vi "WT230.vi"(7 "simulazione":bool, 8 "error in (no error)":errorcluster, 11 "Queue Name":string="WT230_Q") -> (0 "error out":errorcluster, 2 "Stopped":bool)   [LabVIEW 2019]
uses:
  TypeDef/MISURE WT.ctl
  TypeDef/DEVICE NAME.ctl
  <vilib>/Utility/file.llb/Read From Spreadsheet File (string).vi
  <vilib>/Instr/_visa.llb/VISA Configure Serial Port (Instr).vi
  Globals.vi
panel:
  out "String 2":string
  out "error out 3":errorcluster
  out "error out 2":errorcluster
  out "Numeric":i32
  out "String":string
  out "WT230 CONFIG":string[][](array[string])
  out "MISURE WT":T1
  in  "write buffer":string=":MEAS:NORM:ITEM:V:ELEM1 1;ELEM2 1;ELEM3 1;SIGMA 1;:MEAS:NORM:ITEM:A:ELEM1 1;ELEM2 1;ELEM3 1;SIGMA 1;:MEAS:NORM:ITEM:W:ELEM1 1;ELEM2 1;ELEM3 1;SIGMA 1;:MEAS:NORM:ITEM:VA:ELEM1 1;:MEAS:NORM:ITEM:PF:ELEM1 1;:MEAS:NORM:ITEM:PF:SIGMA 1;:MEAS:NORM:ITEM:VHZ:ELEM1 1;"
  out "# elements in queue":i32
  out "Inizialize error":errorcluster
  out "WT230 Settings":string[][](array[string])
  out "LOOP TIME (ms)":u32
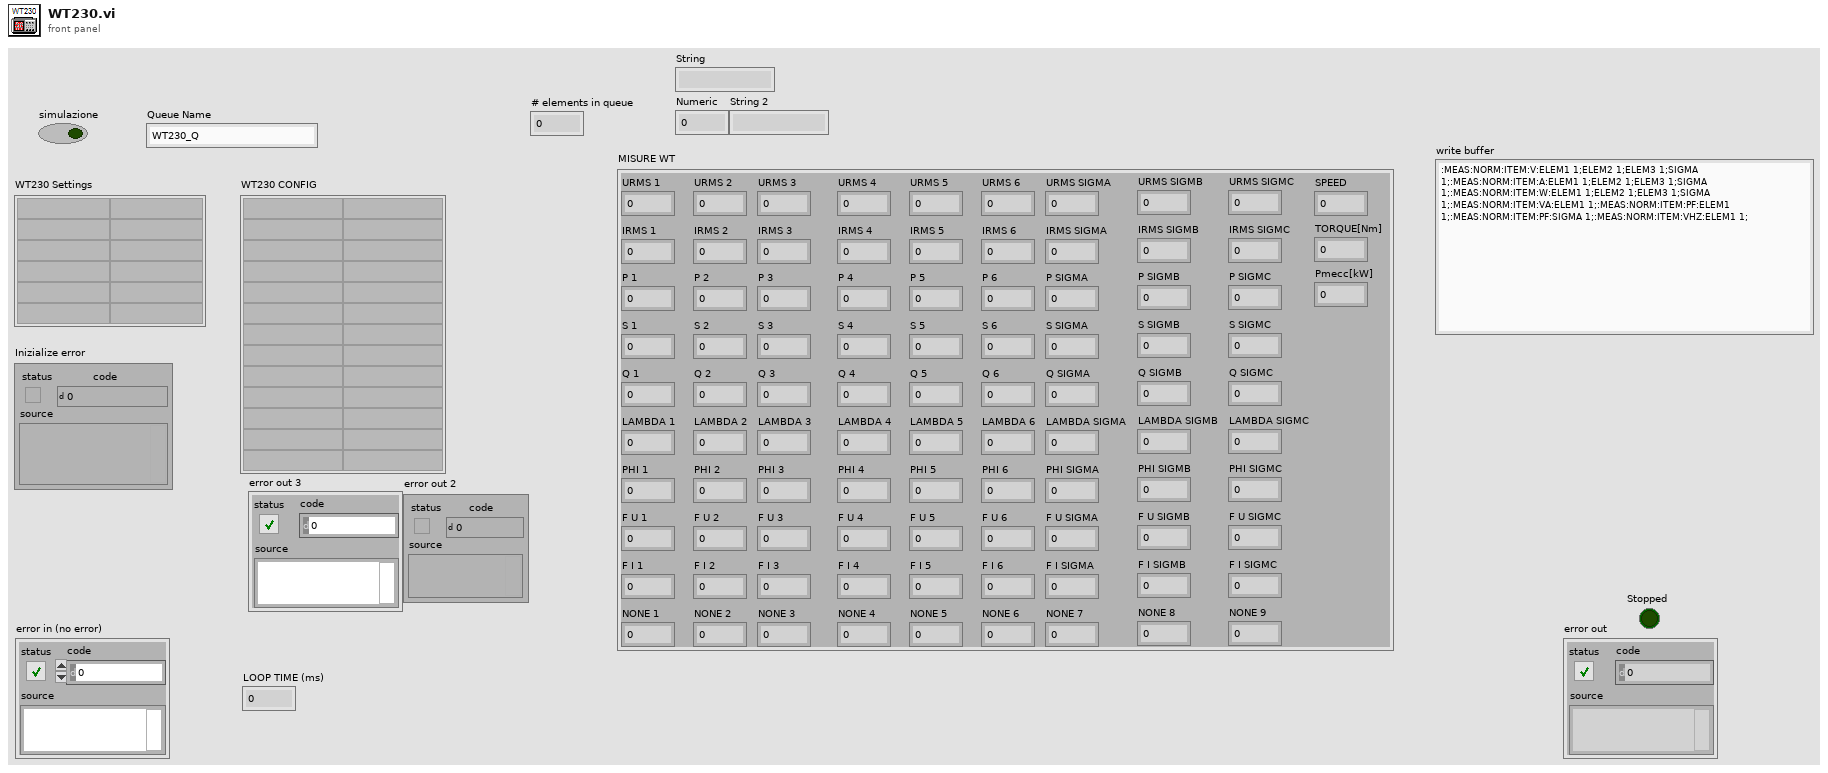
[diagram p1: front panel]
types:
  T1 = typedef "MISURE WT.ctl" = cluster{"URMS 1":dbl, "IRMS 1":dbl, "P 1":dbl, "S 1":dbl, "Q 1":dbl, "LAMBDA 1":dbl, "PHI 1":dbl, "F U 1":dbl, "F I 1":dbl, "NONE 1":dbl, "URMS 2":dbl, "IRMS 2":dbl, "P 2":dbl, "S 2":dbl, "Q 2":dbl, "LAMBDA 2":dbl, "PHI 2":dbl, "F U 2":dbl, "F I 2":dbl, "NONE 2":dbl, "URMS 3":dbl, "IRMS 3":dbl, "P 3":dbl, "S 3":dbl, "Q 3":dbl, "LAMBDA 3":dbl, "PHI 3":dbl, "F U 3":dbl, "F I 3":dbl, "NONE 3":dbl, "URMS 4":dbl, "IRMS 4":dbl, "P 4":dbl, "S 4":dbl, "Q 4":dbl, "LAMBDA 4":dbl, "PHI 4":dbl, "F U 4":dbl, "F I 4":dbl, "NONE 4":dbl, "URMS 5":dbl, "IRMS 5":dbl, "P 5":dbl, "S 5":dbl, "Q 5":dbl, "LAMBDA 5":dbl, "PHI 5":dbl, "F U 5":dbl, "F I 5":dbl, "NONE 5":dbl, "URMS 6":dbl, "IRMS 6":dbl, "P 6":dbl, "S 6":dbl, "Q 6":dbl, "LAMBDA 6":dbl, "PHI 6":dbl, "F U 6":dbl, "F I 6":dbl, "NONE 6":dbl, "URMS SIGMA":dbl, "IRMS SIGMA":dbl, "P SIGMA":dbl, "S SIGMA":dbl, "Q SIGMA":dbl, "LAMBDA SIGMA":dbl, "PHI SIGMA":dbl, "F U SIGMA":dbl, "F I SIGMA":dbl, "NONE 7":dbl, "URMS SIGMB":dbl, "IRMS SIGMB":dbl, "P SIGMB":dbl, "S SIGMB":dbl, "Q SIGMB":dbl, "LAMBDA SIGMB":dbl, "PHI SIGMB":dbl, "F U SIGMB":dbl, "F I SIGMB":dbl, "NONE 8":dbl, "URMS SIGMC":dbl, "IRMS SIGMC":dbl, "P SIGMC":dbl, "S SIGMC":dbl, "Q SIGMC":dbl, "LAMBDA SIGMC":dbl, "PHI SIGMC":dbl, "F U SIGMC":dbl, "F I SIGMC":dbl, "NONE 9":dbl, "SPEED":dbl, "TORQUE[Nm]":dbl, "Pmecc[kW]":dbl}
  T2 = typedef "DEVICE NAME.ctl" = enum16{"WATTMETRO", "APLUS", "PLC BANCO 1", "PLC RACK", "PLC BANCO 2", "PS", "NI cDAQ", "RESISTOMAT"}
  T3 = cluster{"Array of elements":cluster{"String":string, "variant":variant}[], "Single element":cluster{"String":string, "variant":variant}, "enque at\nopposite end (F)":bool, "no replications (F)":bool}
  T4 = cluster{"Measure Value[0]":dbl, "Measure Value[1]":dbl, "Measure Value[2]":dbl, "Measure Value[3]":dbl, "Measure Value[4]":dbl, "Measure Value[5]":dbl, "Measure Value[6]":dbl, "Measure Value[7]":dbl, "Measure Value[8]":dbl, "Measure Value[9]":dbl, "Measure Value[10]":dbl, "Measure Value[11]":dbl, "Measure Value[12]":dbl, "Measure Value[13]":dbl, "Measure Value[14]":dbl, "Measure Value[15]":dbl, "Measure Value[16]":dbl, "Measure Value[17]":dbl, "Measure Value[18]":dbl, "Measure Value[19]":dbl, "Measure Value[20]":dbl, "Measure Value[21]":dbl, "Measure Value[22]":dbl, "Measure Value[23]":dbl, "Measure Value[24]":dbl, "Measure Value[25]":dbl, "Measure Value[26]":dbl, "Measure Value[27]":dbl, "Measure Value[28]":dbl, "Measure Value[29]":dbl, "Measure Value[30]":dbl, "Measure Value[31]":dbl, "Measure Value[32]":dbl, "Measure Value[33]":dbl, "Measure Value[34]":dbl, "Measure Value[35]":dbl, "Measure Value[36]":dbl, "Measure Value[37]":dbl, "Measure Value[38]":dbl, "Measure Value[39]":dbl, "Measure Value[40]":dbl, "Measure Value[41]":dbl, "Measure Value[42]":dbl, "Measure Value[43]":dbl, "Measure Value[44]":dbl, "Measure Value[45]":dbl, "Measure Value[46]":dbl, "Measure Value[47]":dbl, "Measure Value[48]":dbl, "Measure Value[49]":dbl, "Measure Value[50]":dbl, "Measure Value[51]":dbl, "Measure Value[52]":dbl, "Measure Value[53]":dbl, "Measure Value[54]":dbl, "Measure Value[55]":dbl, "Measure Value[56]":dbl, "Measure Value[57]":dbl, "Measure Value[58]":dbl, "Measure Value[59]":dbl, "Measure Value[60]":dbl, "Measure Value[61]":dbl, "Measure Value[62]":dbl, "Measure Value[63]":dbl, "Measure Value[64]":dbl, "Measure Value[65]":dbl, "Measure Value[66]":dbl, "Measure Value[67]":dbl, "Measure Value[68]":dbl, "Measure Value[69]":dbl, "Measure Value[70]":dbl, "Measure Value[71]":dbl, "Measure Value[72]":dbl, "Measure Value[73]":dbl, "Measure Value[74]":dbl, "Measure Value[75]":dbl, "Measure Value[76]":dbl, "Measure Value[77]":dbl, "Measure Value[78]":dbl, "Measure Value[79]":dbl, "Measure Value[80]":dbl, "Measure Value[81]":dbl, "Measure Value[82]":dbl, "Measure Value[83]":dbl, "Measure Value[84]":dbl, "Measure Value[85]":dbl, "Measure Value[86]":dbl, "Measure Value[87]":dbl, "Measure Value[88]":dbl, "Measure Value[89]":dbl, "Measure Value[90]":dbl, "Measure Value[91]":dbl, "Measure Value[92]":dbl}
  T5 = enum32{"Invalid", "Standard", "Closed", "Hidden", "Minimized", "Maximized"}
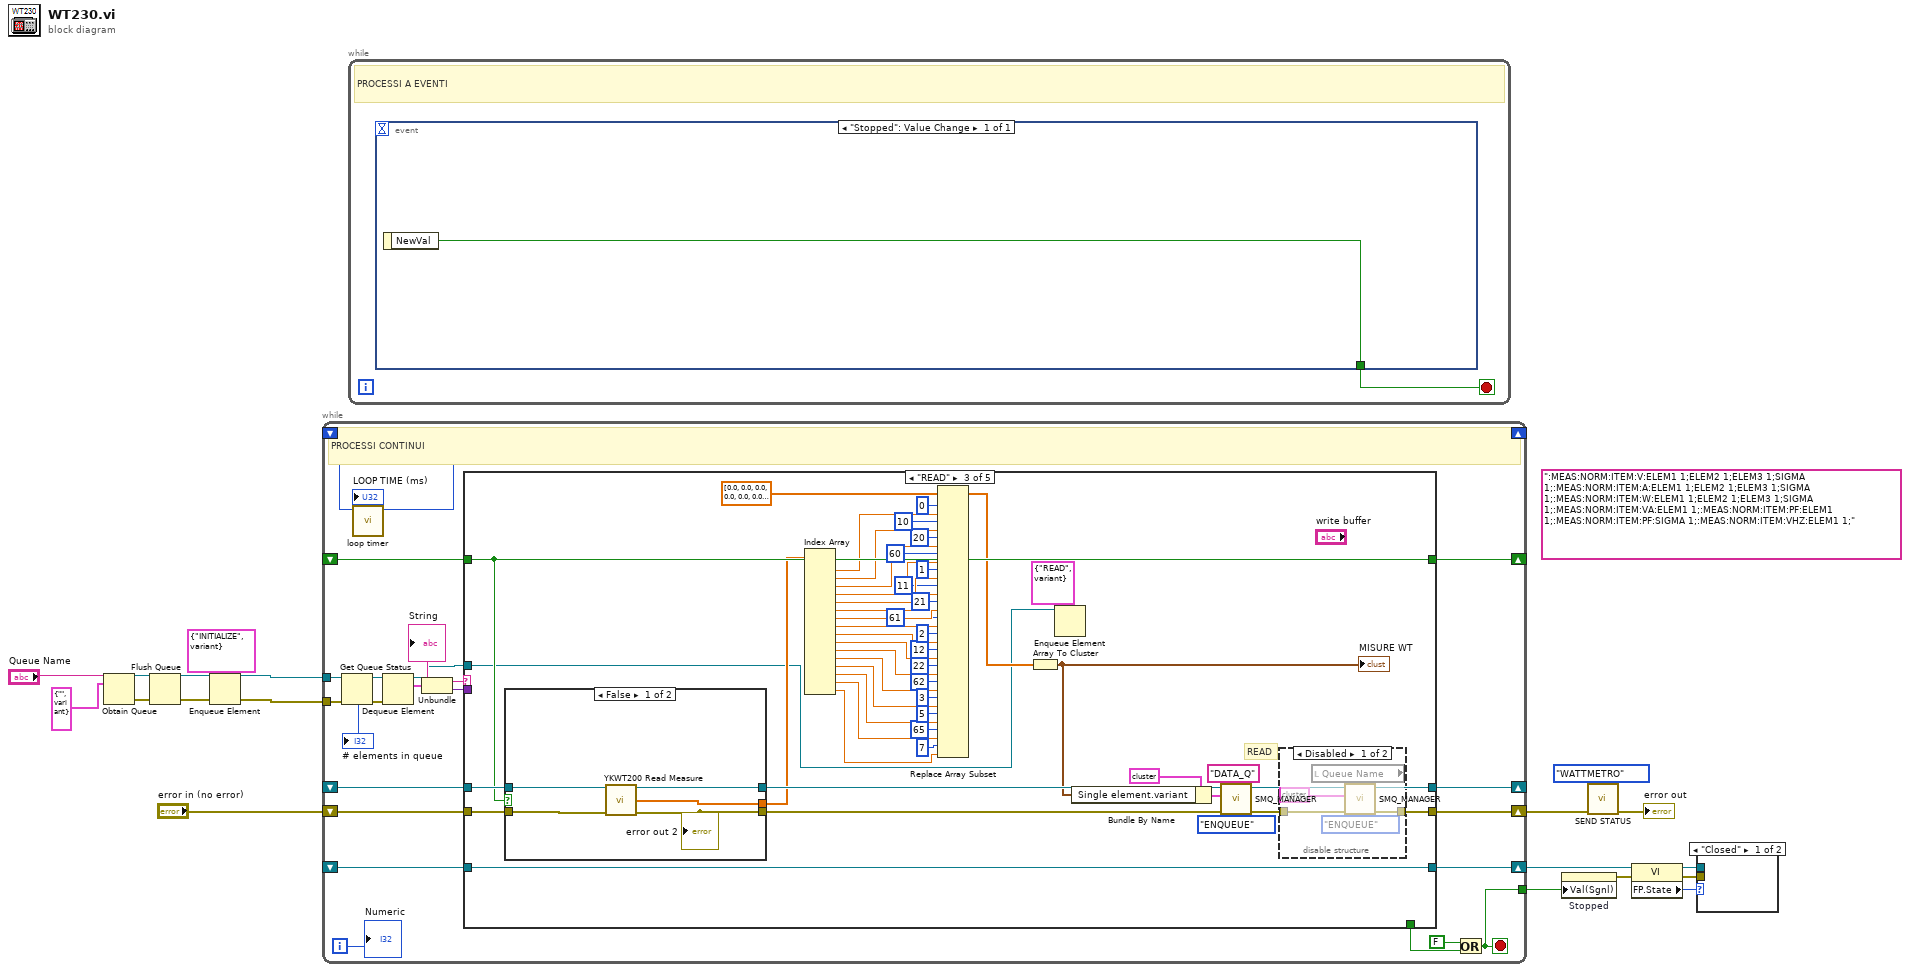
[diagram p0: block diagram]
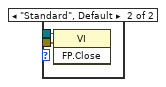
[diagram p2: hidden frame]
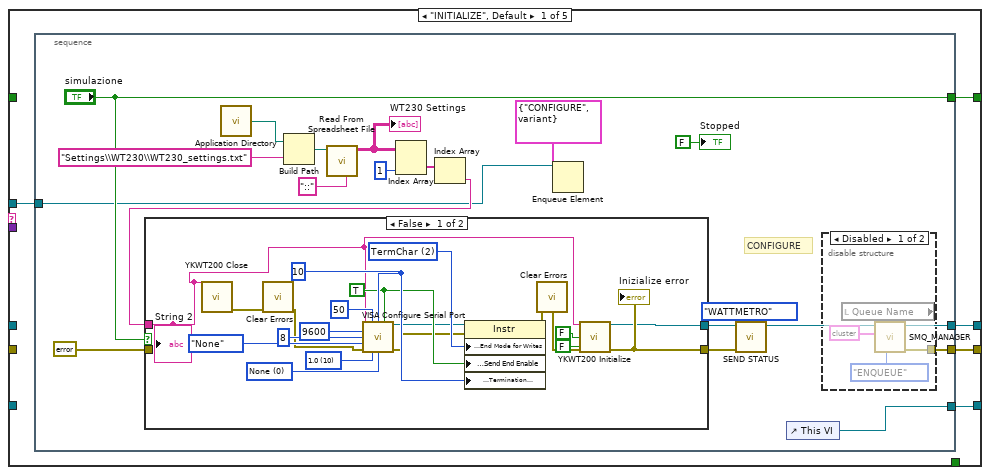
[diagram p3: hidden frame]
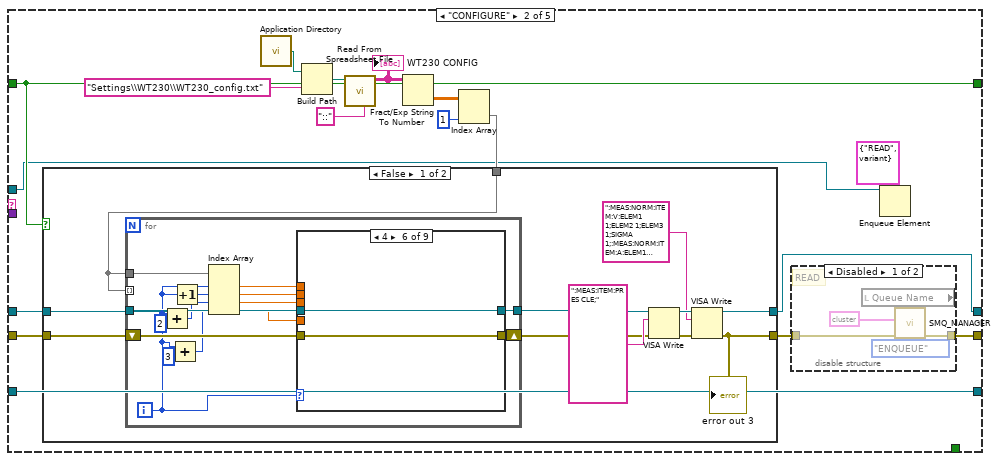
[diagram p6: hidden frame]
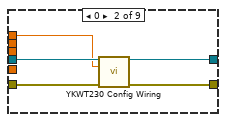
[diagram p9: hidden frame]
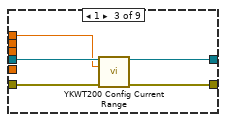
[diagram p10: hidden frame]
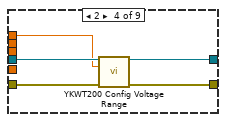
[diagram p11: hidden frame]
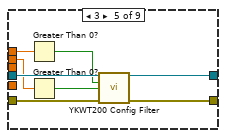
[diagram p12: hidden frame]
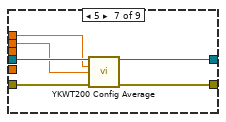
[diagram p13: hidden frame]
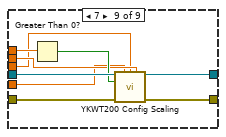
[diagram p15: hidden frame]
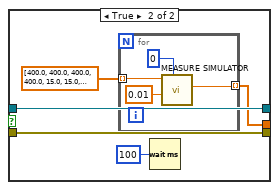
[diagram p18: hidden frame]
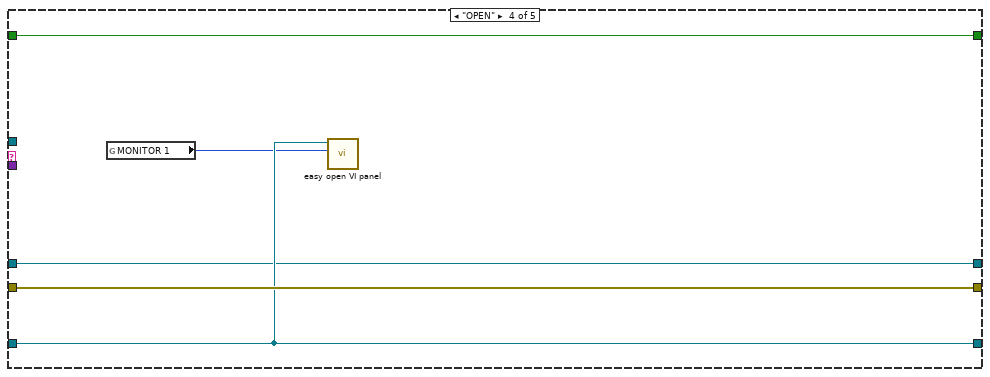
[diagram p19: hidden frame]
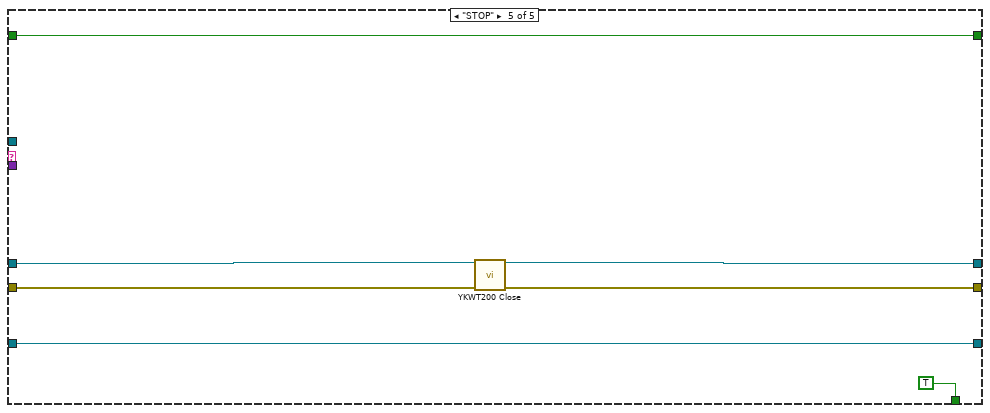
[diagram p20: hidden frame]
diagram:
  (unwired) ":MEAS:NORM:ITEM:V:ELEM1 1;ELEM2 1;ELEM3 1;SIGMA 1;:MEAS:NORM:ITEM:A:ELEM1 1;ELEM2 1;ELEM3 1;SIGMA 1;:MEAS:NORM:ITEM:W:ELEM1 1;ELEM2 1;ELEM3 1;SIGMA 1;:MEAS:NORM:ITEM:VA:ELEM1 1;:MEAS:NORM:ITEM:PF:ELEM1 1;:MEAS:NORM:ITEM:PF:SIGMA 1;:MEAS:NORM:ITEM:VHZ:ELEM1 1;" ("write buffer")
  n1 = Obtain Queue(name (unnamed)="Queue Name", element data type=cluster{"String":string, "variant":variant} {"String"="", "variant"=variant} ("element")) -> (queue out=w8:refnum<queue>, error out=w7:errorcluster)  [unwired: 3 in, 1 out]
  n2 = Flush Queue(queue=w8, error in (no error)=w7) -> (queue out=w5:refnum<queue>, error out=w4:errorcluster)  [unwired: 1 out]
  n3 = Enqueue Element(queue=w5, element=cluster{"String":string, "variant":variant} {"String"="INITIALIZE", "variant"=variant}, error in (no error)=w4) -> (queue out=w10:refnum<queue>, error out=w9:errorcluster)  [unwired: 1 in, 1 out]
  n4 = while {
    shift-right: [w43] -> _
    shift-left: _ -> [w42]
    shift-right: [w40] -> w13
    shift-left: _ -> [w39]
    shift-right: [w36] -> w2
    shift-left: "error in (no error)" -> [w38]
    tunnel: w10 -> [w27]
    tunnel: w9 -> [w26]
    tunnel: [w33] -> w16
    shift-right: [w31] -> _
    shift-left: _ -> [w30]
    shift-right: [w29] -> _
    shift-left: _ -> [w28]
    i -> [w20]
    stop <- w33 stop-if-true
    # "PROCESSI CONTINUI"
    n5 = Get Queue Status(queue=w27, error in (no error)=w26) -> (queue out=w24:refnum<queue>, error out=w25:errorcluster, # elements in queue=→"# elements in queue":i32)  [unwired: 1 in, 5 out]
    n6 = call <userlib>:"loop timer.vi"("millisecond timer IN"=w42) -> ("millisecond timer OUT"=w43:u32, "LOOP TIME (ms)"=→"LOOP TIME (ms)":u32)  [unwired: 9 in]
    n7 = Dequeue Element(queue=w24, error in (no error)=w25) -> (queue out=w21:refnum<queue>, element=w35:cluster{"String":string, "variant":variant})  [unwired: 1 in, 2 out]
    n8 = Unbundle(w35) -> ("String"=w32:string, "variant"=w34:variant)
    "String" <- w32
    n9 = case shown="\"READ\"" w32 {
      tunnel: [_ _ _ _ TRUE] -> w37
      tunnel: [w48 w108 w235 w258 w264] -> w40
      tunnel: w39 -> [_ w108 w235 w258 w264]
      tunnel: w38 -> [_ w105 w233 w259 w263]
      tunnel: [w46 w107 w234 w259 w262] -> w36
      tunnel: w34 -> [_ _ _ _ _]
      tunnel: [w47 w92 w231 w257 w261] -> w31
      tunnel: w30 -> [_ w106 w232 w257 w261]
      tunnel: [w45 w103 w224 w256 w260] -> w29
      tunnel: w28 -> [_ w103 w224 w256 w260]
      tunnel: w21 -> [w44 w93 w187 _ _]
      frame "INITIALIZE", Default {
        n10 = stacked-sequence {
          tunnel: [w66] -> w48
          tunnel: [w54] -> w47
          tunnel: [w57] -> w46
          tunnel: ["simulazione"] -> w45
          tunnel: w44 -> [w50]
          frame #0 {
            # "CONFIGURE"
            n11 = call <vilib>:"Application Directory.vi"() -> ("Application Directory"=w64:path)
            n12 = Build Path(base path=w64, name or relative path="Settings\\WT230\\WT230_settings.txt") -> (appended path=w62:path)
            n13 = call-poly <vilib>:"Read From Spreadsheet File.vi"("delimiter (\\t)"="::" ("delimiter (\\t)"), "file path (dialog if empty)"=w62) -> ("all rows"=w61:string[][])  [unwired: 5 in, 4 out]
            "WT230 Settings" <- w61
            n14 = Index Array(array=w61, index (col)=1 ("disabled index (col)")) -> (element=w59:string[])  [unwired: 1 in]
            n15 = Index Array(array=w59) -> (element=w51:string)  [unwired: 1 in]
            n16 = case shown="False" "simulazione" {
              tunnel: errorcluster {"status"=FALSE, "code"=0, "source"=""} ("error in (no error)") -> [_ w91]
              tunnel: [w90 w91] -> w55
              tunnel: [w89 _] -> w54
              tunnel: w51 -> [w71 _]
              frame False {
                w79 = u16 10 items=["1.0"=10, "1.5"=15, "2.0"=20] ("stop bits (10: 1 bit)")
                w78 = u16 0 items=["None", "XON/XOFF", "RTS/CTS", "XON/XOFF & RTS/CTS", "DTR/DSR", "XON/XOFF & DTR/DSR"] ("flow control (0:none)")
                w77 = TRUE ("Enable Termination\nChar (T)")
                w85 = u8 10 ("termination char\n(0xA = '\\n' = LF)")
                w87 = u16 2 items=["None", "LastBit", "TermChar", "Break"] ("Serial Settings:Serial End Mode for Writes")
                n17 = call <instrlib>:"YKWT200 Close.vi"("VISA session"=w71) -> ("error out"=w83:errorcluster)  [unwired: 14 in]
                n18 = call <vilib>:"Clear Errors.vi"("error in (no error)"=w83) -> ("error out"=w73:errorcluster)  [unwired: 5 in, 1 out]
                n19 = call-poly "VISA Configure Serial Port"("VISA resource name"=w71, "timeout (10sec)"=u32 50, "termination char\n(0xA = '\\n' = LF)"=w85, "Enable Termination\nChar (T)"=w77, "baud rate (9600)"=u32 9600, "data bits (8)"=u16 8, "parity (0:none)"=enum16{"None", "Odd", "Even", "Mark", "Space"}."None", "error in (no error)"=w73, "stop bits (10: 1 bit)"=w79, "flow control (0:none)"=w78) -> ("VISA resource name out"=w76:refnum<visa-resource-name>, "error out"=w75:errorcluster)  [unwired: 4 in]
                n20 = property class="Instr"(reference=w76, error in=w75, "Serial Settings:End Mode for Writes"=w87, "Message Based Settings:Send End Enable"=w77, "Message Based Settings:Termination Character"=w85) -> (error out=w86:errorcluster)  [unwired: 1 out]
                n21 = call <vilib>:"Clear Errors.vi"("error in (no error)"=w86) -> ("error out"=w72:errorcluster)  [unwired: 5 in, 1 out]
                n22 = call <instrlib>:"YKWT200 Initialize.vi"("Instrument Descriptor (GPIB::1)"=w71, "ID Query (T: Check)"=FALSE, "Reset (T: Reset)"=FALSE, "error in (no error)"=w72) -> ("VISA session"=w89:refnum<visa-resource-name>, "error out"=w90:errorcluster)  [unwired: 10 in]
                "Inizialize error" <- w90
                "String 2" <- w71
              }
              frame True {
              }
            }
            n23 = Enqueue Element(queue=w50, element=cluster{"String":string, "variant":variant} {"String"="CONFIGURE", "variant"=variant}) -> ()  [unwired: 2 in, 3 out]
            n24 = call "SEND STATUS.vi"("ELEMENT"=DEVICE_NAME."WATTMETRO", "error in (no error)"=w55) -> ()  [unwired: 9 in, 1 out]
            n25 = control-ref of="This VI"() -> (w66:refnum<vi>)
            n26 = disable-structure shown="Disabled" {
              disable-tunnel: [w70 _] -> w57
              frame Disabled {
                n27 = local read "Queue Name"() -> (w68:string)
                n28 = call <userlib>:"SMQ_MANAGER.vi"("Function"=enum16{"INITIALIZE", "ENQUEUE", "STOP ALL"}."ENQUEUE", "Queue name"=w68, "Enqueue cluster"=T3 {"Array of elements"=[], "Single element"={"String"="CONFIGURE", "variant"=variant}, "enque at\nopposite end (F)"=FALSE, "no replications (F)"=FALSE}) -> ("error out"=w70:errorcluster)  [unwired: 8 in]
              }
              frame Enabled {
              }
            }
            "Stopped" <- FALSE ("Stop")
          }
        }
      }
      frame "CONFIGURE" {
        n29 = call <vilib>:"Application Directory.vi"() -> ("Application Directory"=w102:path)
        n30 = Build Path(base path=w102, name or relative path="Settings\\WT230\\WT230_config.txt") -> (appended path=w100:path)
        n31 = call-poly <vilib>:"Read From Spreadsheet File.vi"("delimiter (\\t)"="::" ("delimiter (\\t)"), "file path (dialog if empty)"=w100) -> ("all rows"=w98:string[][])  [unwired: 5 in, 4 out]
        "WT230 CONFIG" <- w98
        n32 = Fract/Exp String To Number(string=w98) -> (number=w97:dbl[][])  [unwired: 3 in, 1 out]
        n33 = Index Array(array=w97, index (col)=1 ("disabled index (col)")) -> (element=w95:dbl[])  [unwired: 1 in]
        n34 = case shown="False" w103 {
          tunnel: w106 -> [w124 w185]
          tunnel: w105 -> [w123 w184]
          tunnel: [w115 w185] -> w92
          tunnel: [w114 w184] -> w104
          tunnel: w95 -> [w122 _]
          frame False {
            n35 = for {
              tunnel: w124 -> [w139]
              tunnel: w122 -> [w137]
              tunnel: w122 -> [_] mode=indexing
              tunnel: [w126] -> w116
              shift-right: [w125] -> w117
              shift-left: w123 -> [w138]
              i -> [w127]
              n36 = Add(x=w127, y=2) -> (x+y=w130:i32)
              n37 = Add(x=w127, y=3) -> (x+y=w128:i32)
              n38 = Increment(x=w127) -> (x+1=w134:i32)
              n39 = Index Array(array=w137, index #1=w127, index #2=w134, index #3=w130, index #4=w128) -> (element #1=w136:dbl, element #2=w135:dbl, element #3=w133:dbl, element #4=w132:dbl)
              n40 = case shown="4" w127 {
                tunnel: w139 -> [w141 w146 w151 w156 w164 w166 w172 w174 w183]
                tunnel: w138 -> [w140 w145 w150 w155 w163 w165 w171 w173 w182]
                tunnel: w136 -> [_ w144 w149 w154 w162 _ w170 _ w181]
                tunnel: w135 -> [_ _ _ _ w160 _ w169 _ w179]
                tunnel: w133 -> [_ _ _ _ _ _ _ _ w178]
                tunnel: w132 -> [_ _ _ _ _ _ _ _ w177]
                tunnel: [w141 w143 w147 w153 w158 w166 w167 w174 w175] -> w126
                tunnel: [w140 w142 w148 w152 w157 w165 w168 w173 w176] -> w125
                frame -1, Default {
                }
                frame 0 {
                  n41 = call <instrlib>:"YKWT230 Config Wiring.vi"("VISA session"=w146, "Wiring (1: 1P3W)"=w144, "error in (no error)"=w145) -> ("dup VISA session"=w143:refnum<visa-resource-name>, "error out"=w142:errorcluster)  [unwired: 11 in]
                }
                frame 1 {
                  n42 = call <instrlib>:"YKWT200 Config Current Range.vi"("VISA session"=w151, "A Range (12: 20A)"=w149, "error in (no error)"=w150) -> ("dup VISA session"=w147:refnum<visa-resource-name>, "error out"=w148:errorcluster)  [unwired: 11 in]
                }
                frame 2 {
                  n43 = call <instrlib>:"YKWT200 Config Voltage Range.vi"("VISA session"=w156, "V Range (6: 600V)"=w154, "error in (no error)"=w155) -> ("dup VISA session"=w153:refnum<visa-resource-name>, "error out"=w152:errorcluster)  [unwired: 11 in]
                }
                frame 3 {
                  n44 = Greater Than 0?(x=w162) -> (x > 0?=w161:bool)
                  n45 = Greater Than 0?(x=w160) -> (x > 0?=w159:bool)
                  n46 = call <instrlib>:"YKWT200 Config Filter.vi"("VISA session"=w164, "Filter (F: OFF)"=w161, "Line Filter (F: OFF)"=w159, "error in (no error)"=w163) -> ("dup VISA session"=w158:refnum<visa-resource-name>, "error out"=w157:errorcluster)  [unwired: 10 in]
                }
                frame 4 {
                }
                frame 5 {
                  n47 = call <instrlib>:"YKWT200 Config Average.vi"("VISA session"=w172, "Average Type (0: OFF)"=w170, "Constant (0: 8)"=w169, "error in (no error)"=w171) -> ("dup VISA session"=w167:refnum<visa-resource-name>, "error out"=w168:errorcluster)  [unwired: 10 in]
                }
                frame 6 {
                }
                frame 7 {
                  n48 = Greater Than 0?(x=w181) -> (x > 0?=w180:bool)
                  n49 = call <instrlib>:"YKWT200 Config Scaling.vi"("VISA session"=w183, "Power Coefficient (1.000)"=w177, "CT Ratio (1.000)"=w178, "PT Ratio (1.000)"=w179, "Scaling (F: OFF)"=w180, "error in (no error)"=w182) -> ("dup VISA session"=w175:refnum<visa-resource-name>, "error out"=w176:errorcluster)  [unwired: 8 in]
                }
              }
            }
            n50 = VISA Write(VISA resource name=w116, write buffer=":MEAS:ITEM:PRES CLE;", error in (no error)=w117) -> (VISA resource name out=w120:refnum<visa-resource-name>, error out=w121:errorcluster)  [unwired: 1 out]
            n51 = VISA Write(VISA resource name=w120, write buffer=":MEAS:NORM:ITEM:V:ELEM1 1;ELEM2 1;ELEM3 1;SIGMA 1;:MEAS:NORM:ITEM:A:ELEM1 1;ELEM2 1;ELEM3 1;SIGMA 1;:MEAS:NORM:ITEM:W:ELEM1 1;ELEM2 1;ELEM3 1;SIGMA 1;:MEAS:NORM:ITEM:VA:ELEM1 1;:MEAS:NORM:ITEM:PF:ELEM1 1;:MEAS:NORM:ITEM:PF:SIGMA 1;:MEAS:NORM:ITEM:VHZ:ELEM1 1;", error in (no error)=w121) -> (VISA resource name out=w115:refnum<visa-resource-name>, error out=w114:errorcluster)  [unwired: 1 out]
            "error out 3" <- w114
          }
          frame True {
          }
        }
        n52 = disable-structure shown="Disabled" {
          disable-tunnel: [w113 _] -> w107
          disable-tunnel: w104 -> [w112 _]
          frame Disabled {
            # "READ"
            n53 = local read "Queue Name"() -> (w110:string)
            n54 = call <userlib>:"SMQ_MANAGER.vi"("Function"=enum16{"INITIALIZE", "ENQUEUE", "STOP ALL"}."ENQUEUE", "Queue name"=w110, "error in (no error)"=w112, "Enqueue cluster"=T3 {"Array of elements"=[], "Single element"={"String"="READ", "variant"=variant}, "enque at\nopposite end (F)"=FALSE, "no replications (F)"=FALSE}) -> ("error out"=w113:errorcluster)  [unwired: 7 in]
          }
          frame Enabled {
          }
        }
        n55 = Enqueue Element(queue=w93, element=cluster{"String":string, "variant":variant} {"String"="READ", "variant"=variant}) -> ()  [unwired: 2 in, 3 out]
      }
      frame "READ" {
        # "READ"
        n56 = case shown="False" w224 {
          tunnel: w233 -> [w245 w249]
          tunnel: w232 -> [w243 w250]
          tunnel: [w242 w250] -> w231
          tunnel: [w244 w249] -> w229
          tunnel: [w241 w247] -> w223
          frame False {
            n57 = call <instrlib>:"YKWT200 Read Measure.vi"("VISA session"=w243, "error in (no error)"=w245) -> ("dup VISA session"=w242:refnum<visa-resource-name>, "Measure Value"=w241:sgl[], "error out"=w244:errorcluster)  [unwired: 10 in, 1 out]
            "error out 2" <- w244
          }
          frame True {
            n58 = for {
              tunnel: dbl[] [400.0, 400.0, 400.0, 400.0, 15.0, 15.0, 15.0, 15.0, 4800.0, 4800.0, 4800.0, 4800.0, 6000.0, 0.8, 0.8, 50.0] -> [w253] mode=indexing
              tunnel: [w251] -> w247 mode=indexing
              n59 = call <userlib>:"MEASURE SIMULATOR.vi"("delay (100)"=u32 0, "precision %"=0.01, "amplitude"=w253) -> ("value"=w251:dbl)  [unwired: 8 in]
            }
            n60 = Wait (ms)(milliseconds to wait=u32 100) -> ()  [unwired: 1 out]
          }
        }
        n61 = Index Array(array=w223) -> (element #1=w220:dbl, element #2=w218:dbl, element #3=w216:dbl, element #4=w214:dbl, element #5=w212:dbl, element #6=w210:dbl, element #7=w208:dbl, element #8=w206:dbl, element #9=w204:dbl, element #10=w202:dbl, element #11=w200:dbl, element #12=w198:dbl, element #13=w196:dbl, element #14=w194:dbl, element #15=w192:dbl, element #16=w190:dbl)  [unwired: 16 in]
        n62 = Replace Array Subset(array=dbl[] [0.0, 0.0, 0.0, 0.0, 0.0, 0.0, 0.0, 0.0, 0.0, 0.0, 0.0, 0.0, 0.0, 0.0, 0.0, 0.0, 0.0, 0.0, 0.0, 0.0, 0.0, 0.0, 0.0, 0.0, 0.0, 0.0, 0.0, 0.0, 0.0, 0.0, 0.0, 0.0, 0.0, 0.0, 0.0, 0.0, 0.0, 0.0, 0.0, 0.0, 0.0, 0.0, 0.0, 0.0, 0.0, 0.0, 0.0, 0.0, 0.0, 0.0, 0.0, 0.0, 0.0, 0.0, 0.0, 0.0, 0.0, 0.0, 0.0, 0.0, 0.0, 0.0, 0.0, 0.0, 0.0, 0.0, 0.0, 0.0, 0.0, 0.0, 0.0, 0.0, 0.0, 0.0, 0.0, 0.0, 0.0, 0.0, 0.0, 0.0, 0.0, 0.0, 0.0, 0.0, 0.0, 0.0, 0.0, 0.0, 0.0, 0.0] ("Measure Value"), new element #1=w220, index #1=0 ("index"), new element #2=w218, index #2=10 ("index"), new element #3=w216, index #3=20 ("index"), new element #4=w214, index #4=60 ("index"), new element #5=w212, index #5=1 ("index"), new element #6=w210, index #6=11 ("index"), new element #7=w208, index #7=21 ("index"), new element #8=w206, index #8=61 ("index"), new element #9=w204, index #9=2 ("index"), new element #10=w202, index #10=12 ("index"), new element #11=w200, index #11=22 ("index"), new element #12=w198, index #12=62 ("index"), new element #13=w196, index #13=3 ("index"), new element #14=w194, index #14=5 ("index"), new element #15=w192, index #15=65 ("index"), new element #16=w190, index #16=7 ("index")) -> (w189:dbl[])
        n63 = Array To Cluster(array=w189) -> (cluster=w188:T4)
        "MISURE WT" <- w188
        n64 = Enqueue Element(queue=w187, element=cluster{"String":string, "variant":variant} {"String"="READ", "variant"=variant}) -> ()  [unwired: 2 in, 3 out]
        n65 = Bundle By Name(cluster=T3 {"Array of elements"=[], "Single element"={"String"="READ WT", "variant"=variant}, "enque at\nopposite end (F)"=FALSE, "no replications (F)"=FALSE} ("Enqueue cluster"), "Single element.variant"=w188) -> (w226:T3)
        n66 = call <userlib>:"SMQ_MANAGER.vi"("Function"=enum16{"INITIALIZE", "ENQUEUE", "STOP ALL"}."ENQUEUE", "Queue name"="DATA_Q", "error in (no error)"=w229, "Enqueue cluster"=w226) -> ("error out"=w228:errorcluster)  [unwired: 7 in]
        n67 = disable-structure shown="Disabled" {
          disable-tunnel: [w240 _] -> w234
          disable-tunnel: w228 -> [w239 _]
          frame Disabled {
            n68 = local read "Queue Name"() -> (w237:string)
            n69 = call <userlib>:"SMQ_MANAGER.vi"("Function"=enum16{"INITIALIZE", "ENQUEUE", "STOP ALL"}."ENQUEUE", "Queue name"=w237, "error in (no error)"=w239, "Enqueue cluster"=T3 {"Array of elements"=[], "Single element"={"String"="READ", "variant"=variant}, "enque at\nopposite end (F)"=FALSE, "no replications (F)"=FALSE}) -> ("error out"=w240:errorcluster)  [unwired: 7 in]
          }
          frame Enabled {
          }
        }
      }
      frame "OPEN" {
        n70 = global read "Globals.vi" "MONITOR 1"() -> (w255:u8)
        n71 = call <userlib>:"easy open VI panel.vi"("Monitor(1)"=w255, "VI in"=w258) -> ()  [unwired: 9 in, 1 out]
      }
      frame "STOP" {
        n72 = call <instrlib>:"YKWT200 Close.vi"("VISA session"=w261, "error in (no error)"=w263) -> ("error out"=w262:errorcluster)  [unwired: 13 in]
      }
    }
    n73 = Or(x=FALSE, y=w37) -> (x .or. y?=w33:bool)
    "Numeric" <- w20
  }
  n74 = while {
    stop <- w266 stop-if-true
    # "PROCESSI A EVENTI"
    n75 = event shown="[0] \"Stopped\": Value Change" {
      selector: _ -> [_]
      dyn-events: _ -> [_]
      timeout: _ -> [_]
      tunnel: [w267] -> w266
      event "Stopped": Value Change {
        n76 = event-data() -> ("NewVal"=w267:bool)  [unwired: 1 in]
      }
    }
  }
  n77 = property on="Stopped" class="Bool (strict)"("Val(Sgnl)"=w16) -> (error out=w12:errorcluster)  [unwired: 2 in, 1 out]
  n78 = call "SEND STATUS.vi"("ELEMENT"=DEVICE_NAME."WATTMETRO", "error in (no error)"=w2) -> ("error out"=→"error out":errorcluster)  [unwired: 9 in]
  n79 = property class="VI"(reference=w13, error in=w12) -> (reference out=w15:refnum<vi>, error out=w11:errorcluster, "FP.State"=w14:T5)
  n80 = case shown="\"Closed\"" w14 {
    tunnel: w15 -> [_ w269]
    tunnel: w11 -> [_ w268]
    frame "Closed" {
    }
    frame "Standard", Default {
      n81 = invoke class="VI" method="FP.Close"(reference=w269, error in=w268) -> ()  [unwired: 1 in, 3 out]
    }
  }
